vi "Translate Raw Description Data.vi"(8 "Error In":errorcluster, 10 "Weather Description Raw Data":T2[](array[typedef]), 11 "Open Weather Session In":refnum<class "Open Weather Session.lvclass">) -> (0 "Error Out":errorcluster, 2 "Weather Data":T1, 3 "Open Weather Session Out":refnum<class "Open Weather Session.lvclass">)   [LabVIEW 2021, in "Open Weather Session.lvclass"]
uses:
  Open Weather Session.lvclass
  Controls/Weather Description Raw Data.ctl
  Public/Controls/Weather Description Data.ctl
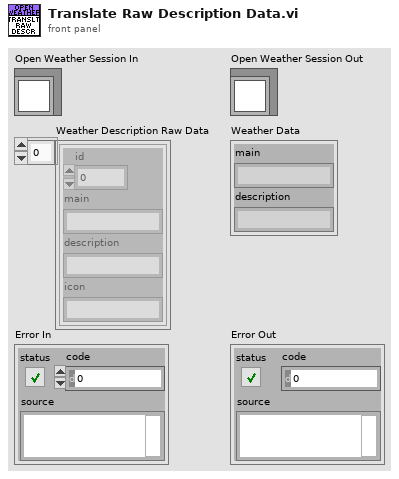
[diagram p1: front panel]
types:
  T1 = typedef "Open Weather Session.lvclass/Weather Description Data.ctl" = cluster{"main":string, "description":string}
  T2 = typedef "Open Weather Session.lvclass/Weather Description Raw Data.ctl" = cluster{"id":u32, "main":string, "description":string, "icon":string}
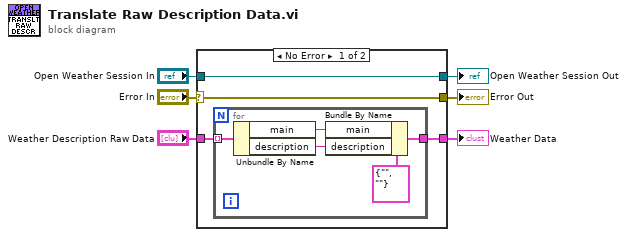
[diagram p0: block diagram]
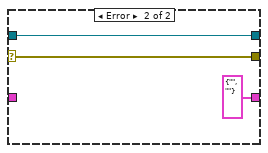
[diagram p2: hidden frame]
diagram:
  n1 = case shown="No Error" "Error In" {
    selector: "Error In" -> [w7 w17]
    tunnel: [w10 w18] -> w6
    tunnel: [w7 w17] -> w5
    tunnel: "Open Weather Session In" -> [w10 w18]
    tunnel: "Weather Description Raw Data" -> [w8 _]
    tunnel: [w9 T1 {"main"="", "description"=""} ("Weather Data")] -> w1
    frame No Error {
      n2 = for {
        tunnel: [w15] -> w9
        tunnel: w8 -> [w14] mode=indexing
        n3 = Unbundle By Name(w14) -> ("main"=w12:string, "description"=w11:string)
        n4 = Bundle By Name(cluster=T1 {"main"="", "description"=""} ("Weather Data"), "main"=w12, "description"=w11) -> (w15:T1)
      }
    }
    frame Error {
    }
  }
  "Open Weather Session Out" <- w6
  "Error Out" <- w5
  "Weather Data" <- w1
